vi "configureOutput.vi"(6 "sofwareTrigger?":bool, 8 "error in (no error)":errorcluster, 9 "Data":variant, 10 "Config":T1, 11 "k3390_AWG in":refnum<class "k3390_AWG.lvclass">) -> (0 "error out":errorcluster, 3 "k3390_AWG out":refnum<class "k3390_AWG.lvclass">)   [LabVIEW 2009, in "Hardware.lvlib" / "Channels.lvlib" / "k3390_AWG.lvclass"]
doc: "Data is an array of varient clusters. One varient cluster per channel.\n\nVariant is a 2D array { {Time, Freq, Amplitude,Phase},...}"
uses:
  k3390_AWG.lvclass
  Generic/DDSOutput.lvclass
  k3390_AWG.lvclass/k3390_AWG.ctl
  <instrlib>/Keithley 3390/Public/Configure/Low Level/Configure Voltage (Amplitude).vi
  <instrlib>/Keithley 3390/Keithley 3390.lvlib
panel:
  out "data (time, freq, amplitude, phase)":dbl[][](array[numeric])
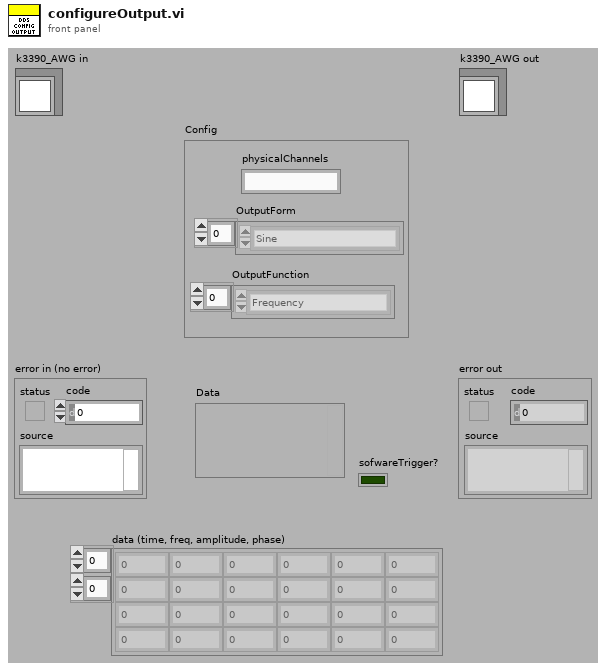
[diagram p1: front panel]
types:
  T1 = cluster{"OutputForm":enum16{"Sine", "Square", "Triangle", "Arbitrary"}[], "OutputFunction":enum16{"Frequency", "Ramp", "Sequence"}[], "physicalChannels":string}
  T2 = enum16{"Sine", "Square", "Ramp", "Pulse", "Noise", "DC", "Arbitrary"}
  T3 = cluster{"data (time, freq, amplitude, phase)":dbl[][]}
  T4 = cluster{"data (time, freq, amplitude, phase)":dbl[][]}[]
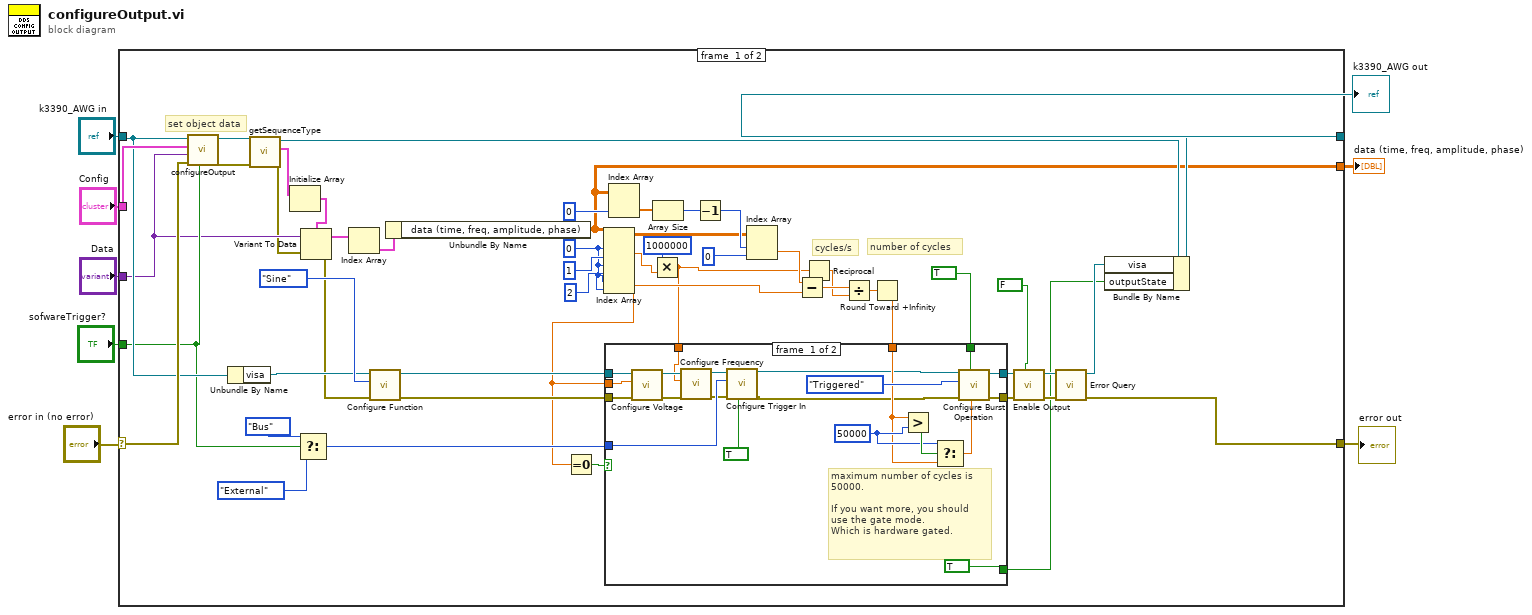
[diagram p0: block diagram]
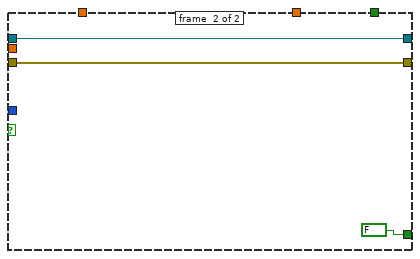
[diagram p2: hidden frame]
diagram:
  n1 = case shown="No Error" "error in (no error)" {
    selector: "error in (no error)" -> [w55 w84]
    tunnel: [w40 w85] -> w7
    tunnel: "k3390_AWG in" -> [w54 w85]
    tunnel: [w23 w84] -> w5
    tunnel: "sofwareTrigger?" -> [w39 _]
    tunnel: "Data" -> [w36 _]
    tunnel: "Config" -> [w56 _]
    tunnel: [w33 _] -> w1
    frame #0 {
      w45 = 0
      # "number of cycles"
      # "cycles/s"
      # "set object data"
      n2 = call-parent "configureOutput.vi"("sofwareTrigger?"=w39, "error in (no error)"=w55, "Data"=w36, "Config"=w56, "DDSOutput in"=w54) -> ("error out"=w57:errorcluster, "DDSOutput out"=w58:refnum<class "k3390_AWG.lvclass">)  [unwired: 5 in]
      n3 = Unbundle By Name(w54) -> ("visa"=w14:refnum<visa-resource-name>)
      n4 = call "getSequenceType.vi"("error in (no error)"=w57, "DDSOutput in"=w58) -> ("error out"=w35:errorcluster, "Sequence"=w59:T3, "DDSOutput out"=w41:refnum<class "k3390_AWG.lvclass">)  [unwired: 7 in]
      n5 = Initialize Array(w59) -> (w37:T4)  [unwired: 1 in]
      n6 = Select(t=enum16{"Immediate", "External", "Bus"}."Bus" ("Trigger Source (0:Immediate)"), s=w39, f=enum16{"Immediate", "External", "Bus"}."External" ("Trigger Source (0:Immediate)")) -> (s? t:f=w22:enum16{"Immediate", "External", "Bus"})
      n7 = Variant To Data(error in=w35, Variant=w36, type=w37) -> (error out=w13:errorcluster, data=w34:T4)
      n8 = Index Array(array=w34) -> (element=w53:T3)  [unwired: 1 in]
      n9 = call <instrlib>:"Configure Function.vi"("error in (no error)"=w13, "Function (Sine)"=T2."Sine", "VISA resource name"=w14) -> ("error out"=w15:errorcluster, "VISA resource name out"=w16:refnum<visa-resource-name>)  [unwired: 7 in]
      n10 = Unbundle By Name(w53) -> ("data (time, freq, amplitude, phase)"=w33:dbl[][])
      n11 = Index Array(array=w33, index (row) #1=w45, index (col) #1=1 ("disabled index (col)"), index (row) #2=w45, index (col) #2=2, index (row) #3=w45, index (col) #3=w45) -> (element #1=w30:dbl, element #2=w10:dbl, element #3=w43:dbl)
      n12 = Equal To 0?(x=w10) -> (x = 0?=w11:bool)
      n13 = Index Array(array=w33, index (col)=0) -> (element=w50:dbl[])  [unwired: 1 in]
      n14 = Multiply(x=1000000, y=w30) -> (x*y=w12:dbl)
      n15 = Array Size(array=w50) -> (size(s)=w48:i32)
      n16 = Decrement(x=w48) -> (x-1=w46:i32)
      n17 = Index Array(array=w33, index (row)=w46, index (col)=0 ("disabled index (col)")) -> (element=w44:dbl)
      n18 = Subtract(x=w44, y=w43) -> (x-y=w32:dbl)
      n19 = Reciprocal(x=w12) -> (1/x=w29:dbl)
      n20 = Divide(x=w32, y=w29) -> (x/y=w42:dbl)
      n21 = Round Toward +Infinity(x=w42) -> (ceil(x): smallest int >= x=w28:dbl)
      n22 = case shown="False" w11 {
        tunnel: w28 -> [w77 _]
        tunnel: [w74 w83] -> w27
        tunnel: TRUE ("Enable Burst Operation (Enable)") -> [w72 _]
        tunnel: w22 -> [w70 _]
        tunnel: [w69 w82] -> w20
        tunnel: w16 -> [w68 w83]
        tunnel: w15 -> [w67 w82]
        tunnel: w12 -> [w62 _]
        tunnel: w10 -> [w61 _]
        tunnel: [TRUE FALSE] -> w9
        frame #0 {
          w78 = 50000
          # "maximum number of cycles is\n50000. \n\nIf you want more, you should\nuse the gate mode.\nWhich is hardware gated."
          n23 = call-poly <instrlib>:"Configure Voltage.vi"("error in (no error)"=w67, "Amplitude (1.00 Vpp)"=w61, "VISA resource name"=w68) -> ("error out"=w65:errorcluster, "VISA resource name out"=w66:refnum<visa-resource-name>)  [unwired: 7 in]
          n24 = call <instrlib>:"Configure Frequency.vi"("error in (no error)"=w65, "Frequency (1000 Hz)"=w62, "VISA resource name"=w66) -> ("error out"=w64:errorcluster, "VISA resource name out"=w63:refnum<visa-resource-name>)  [unwired: 7 in]
          n25 = call <instrlib>:"Configure Trigger In.vi"("error in (no error)"=w64, "External Trigger Slope (T: Positive)"=TRUE, "Trigger Source (0:Immediate)"=w70, "VISA resource name"=w63) -> ("error out"=w75:errorcluster, "VISA resource name out"=w76:refnum<visa-resource-name>)  [unwired: 6 in]
          n26 = Greater?(x=w77, y=w78) -> (0:w79:bool)
          n27 = Select(t=w78, s=w79, f=w77) -> (s? t:f=w71:dbl)
          n28 = call <instrlib>:"Configure Burst Operation.vi"("Burst Count (1)"=w71, "Enable Burst Operation (Enable)"=w72, "error in (no error)"=w75, "Burst Mode (Triggered)"=enum16{"Triggered", "Gated"}."Triggered", "VISA resource name"=w76) -> ("error out"=w69:errorcluster, "VISA resource name out"=w74:refnum<visa-resource-name>)  [unwired: 5 in]
        }
        frame #1 {
        }
      }
      n29 = call <instrlib>:"Enable Output.vi"("Enable Output (T: Enable)"=FALSE, "error in (no error)"=w20, "VISA resource name"=w27) -> ("error out"=w19:errorcluster, "VISA resource name out"=w21:refnum<visa-resource-name>)  [unwired: 7 in]
      n30 = call <instrlib>:"Error Query.vi"("error in (no error)"=w19, "VISA resource name"=w21) -> ("error out"=w23:errorcluster, "VISA resource name out"=w24:refnum<visa-resource-name>)  [unwired: 6 in, 2 out]
      n31 = Bundle By Name(cluster=w41, "visa"=w24, "outputState"=w9) -> (w40:refnum<class "k3390_AWG.lvclass">)
    }
    frame #1 {
    }
  }
  "error out" <- w5
  "k3390_AWG out" <- w7
  "data (time, freq, amplitude, phase)" <- w1
